vi "find lookahead point.vi"(6 "Lookahead Distance":dbl=4000.0, 11 "Path Data":T1={"Path"=[], "Target Velocities"=[], "Robot Location"=[], "Relative Robot Angle (rad)"=0.0, "Curvature"=0.0, "Lookahead Point"=[3064.399009129367, 18229.833030071386], "Lookahead Index"=8.422809037111724, "Closest Point"=[], "Closest Point Index"=0, "Left Velocity"=0.0, "Right Velocity"=0.0, "Left Encoder Vel"=0, "Right Encoder Vel"=0, "Left Encoder Pos"=0, "Right Encoder Pos"=0, "Inital Robot Angle (deg)"=0.0}) -> (3 "Path Data":T1={"Path"=[], "Target Velocities"=[], "Robot Location"=[], "Relative Robot Angle (rad)"=0.0, "Curvature"=0.0, "Lookahead Point"=[3064.399009129367, 18229.833030071386], "Lookahead Index"=8.422809037111724, "Closest Point"=[], "Closest Point Index"=0, "Left Velocity"=0.0, "Right Velocity"=0.0, "Left Encoder Vel"=0, "Right Encoder Vel"=0, "Left Encoder Pos"=0, "Right Encoder Pos"=0, "Inital Robot Angle (deg)"=0.0})   [LabVIEW 2018]
uses:
  path data.ctl
panel:
  out "a":dbl
  out "Lookahead Index":dbl=8.422809037111724
  out "Lookahead Point":dbl[](array[numeric])=[3064.399009129367, 18229.833030071386]
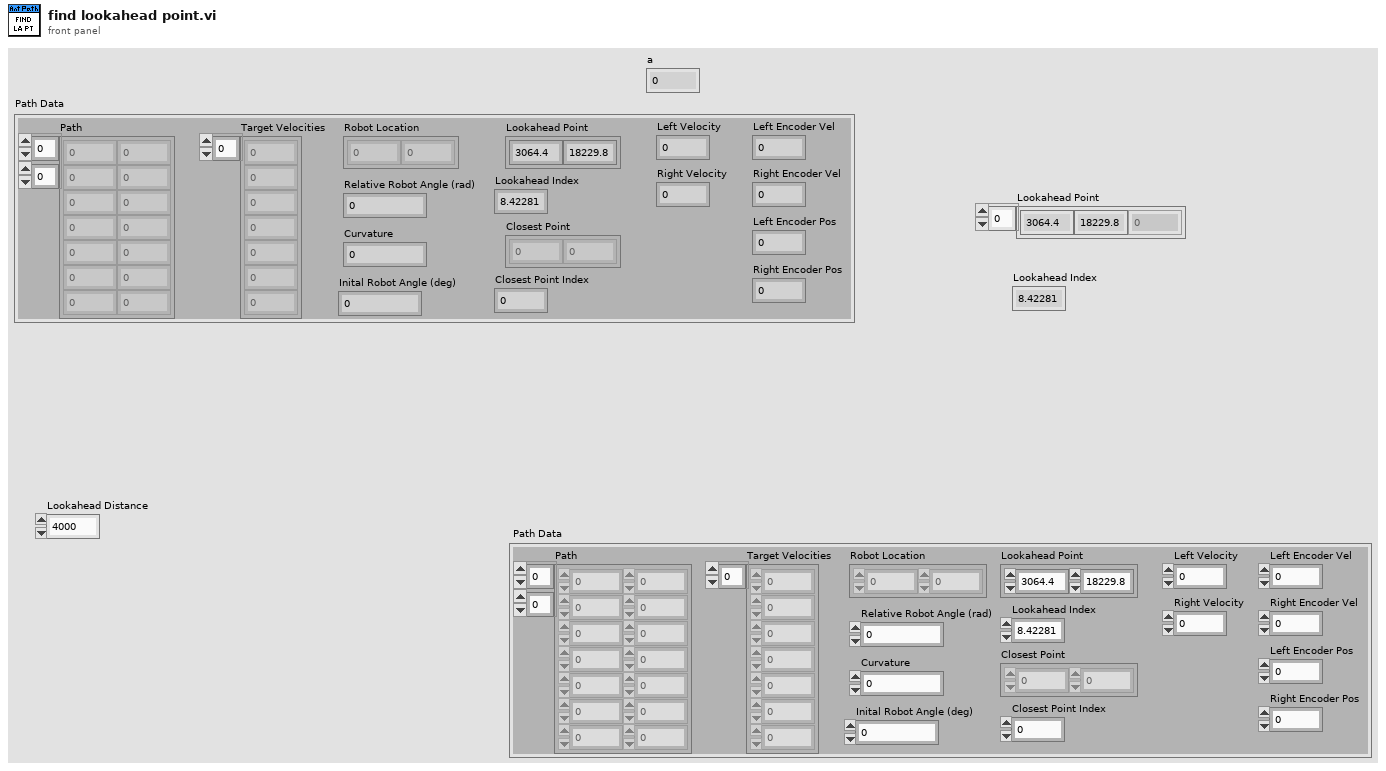
[diagram p1: front panel]
types:
  T1 = typedef "path data.ctl" = cluster{"Path":dbl[][], "Target Velocities":dbl[], "Robot Location":dbl[], "Relative Robot Angle (rad)":dbl, "Curvature":dbl, "Lookahead Point":dbl[], "Lookahead Index":dbl, "Closest Point":dbl[], "Closest Point Index":i32, "Left Velocity":dbl, "Right Velocity":dbl, "Left Encoder Vel":i32, "Right Encoder Vel":i32, "Left Encoder Pos":i32, "Right Encoder Pos":i32, "Inital Robot Angle (deg)":dbl}
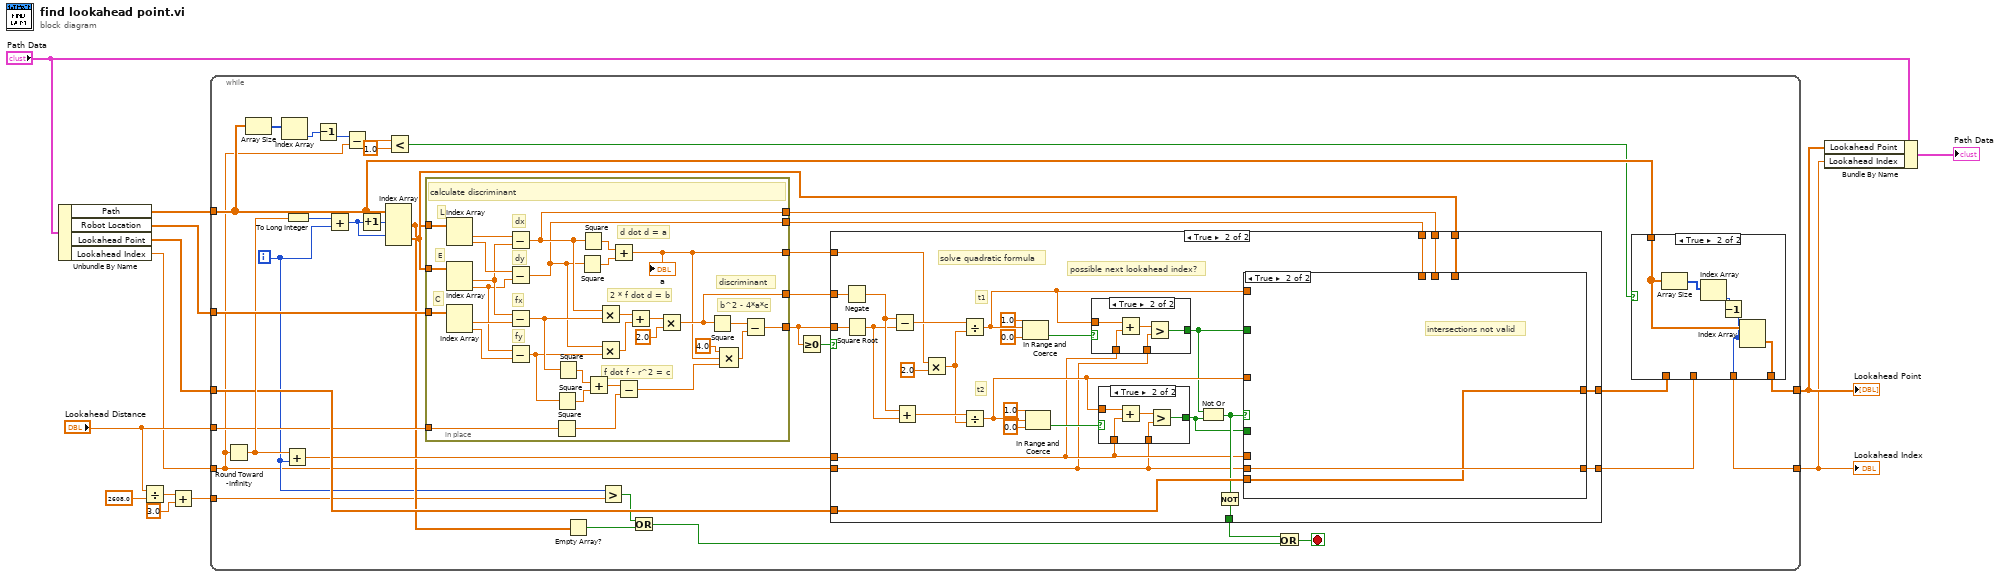
[diagram p0: block diagram]
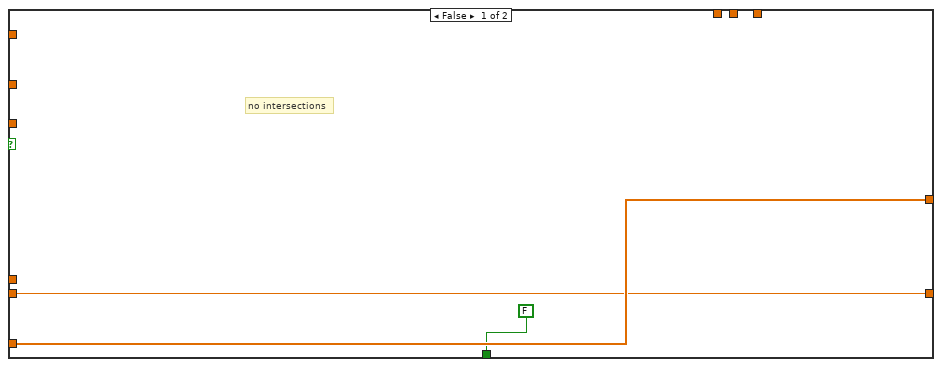
[diagram p3: hidden frame]
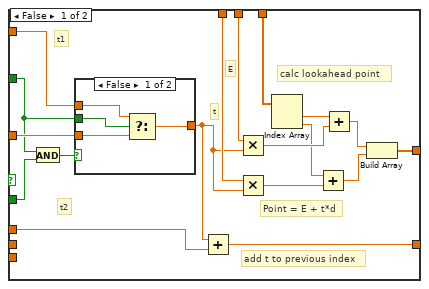
[diagram p4: hidden frame]
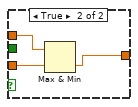
[diagram p5: hidden frame]
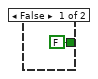
[diagram p6: hidden frame]
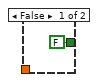
[diagram p7: hidden frame]
diagram:
  n1 = Unbundle By Name("Path Data") -> ("Path"=w4:dbl[][], "Robot Location"=w3:dbl[], "Lookahead Point"=w2:dbl[], "Lookahead Index"=w1:dbl)
  n2 = Divide(x="Lookahead Distance", y=2608.0) -> (x/y=w11:dbl)
  n3 = Add(x=w11, y=3.0) -> (x+y=w9:dbl)
  n4 = while {
    tunnel: w3 -> [w48]
    tunnel: "Lookahead Distance" -> [w39]
    tunnel: w4 -> [w25]
    tunnel: w1 -> [w23]
    tunnel: w2 -> [w41]
    tunnel: [w18] -> w6
    tunnel: [w16] -> w5
    tunnel: w9 -> [w27]
    i -> [w28]
    stop <- w37 stop-if-true
    n5 = Round Toward -Infinity(1:w23) -> (0:w42:dbl)
    n6 = Array Size(array=w25) -> (size(s)=w24:i32[])
    n7 = Index Array(array=w24) -> (element=w15:i32)  [unwired: 1 in]
    n8 = Add(x=w42, y=w28) -> (x+y=w35:dbl)
    n9 = To Long Integer(number=w42) -> (32bit integer=w40:i32)
    n10 = Decrement(x=w15) -> (x-1=w14:i32)
    n11 = Add(x=w40, y=w28) -> (x+y=w34:i32)
    n12 = Subtract(x=w14, y=w23) -> (x-y=w22:dbl)
    n13 = Increment(x=w34) -> (x+1=w32:i32)
    n14 = Index Array(array=w25, index (row) #1=w32, index (row) #2=w34) -> (element #1=w31:dbl[], element #2=w33:dbl[])  [unwired: 2 in]
    n15 = Less?(x=w22, y=1.0) -> (x < y?=w20:bool)
    n16 = in-place {
      in-place-border: w48 -> [w86]
      in-place-border: w39 -> [w69]
      in-place-border: [w62] -> w47
      in-place-border: [w61] -> w46
      in-place-border: [w60] -> w45
      in-place-border: [w59] -> w44
      in-place-border: [w58] -> w43
      in-place-border: w31 -> [w57]
      in-place-border: w33 -> [w56]
      # "C"
      # "E"
      # "L"
      # "calculate discriminant"
      # "b^2 - 4*a*c"
      # "discriminant"
      # "f dot f - r^2 = c"
      # "2 * f dot d = b"
      # "d dot d = a"
      # "fy"
      # "dy"
      # "fx"
      # "dx"
      n17 = Index Array(array=w57) -> (element #1=w85:dbl, element #2=w84:dbl)  [unwired: 2 in]
      n18 = Index Array(array=w56) -> (element #1=w83:dbl, element #2=w81:dbl)  [unwired: 2 in]
      n19 = Index Array(array=w86) -> (element #1=w82:dbl, element #2=w80:dbl)  [unwired: 2 in]
      n20 = Subtract(x=w85, y=w83) -> (x-y=w60:dbl)
      n21 = Subtract(x=w84, y=w81) -> (x-y=w59:dbl)
      n22 = Subtract(x=w83, y=w82) -> (x-y=w73:dbl)
      n23 = Subtract(x=w81, y=w80) -> (x-y=w72:dbl)
      n24 = Square(x=w69) -> (x^2=w68:dbl)
      n25 = Square(x=w72) -> (x^2=w70:dbl)
      n26 = Square(x=w73) -> (x^2=w71:dbl)
      n27 = Square(x=w59) -> (x^2=w79:dbl)
      n28 = Square(x=w60) -> (x^2=w78:dbl)
      n29 = Add(x=w71, y=w70) -> (x+y=w67:dbl)
      n30 = Multiply(x=w60, y=w73) -> (x*y=w77:dbl)
      n31 = Multiply(x=w59, y=w72) -> (x*y=w76:dbl)
      n32 = Add(x=w78, y=w79) -> (x+y=w58:dbl)
      "a" <- w58
      n33 = Subtract(x=w67, y=w68) -> (x-y=w64:dbl)
      n34 = Add(x=w77, y=w76) -> (x+y=w75:dbl)
      n35 = Multiply(x=w75, y=2.0) -> (x*y=w62:dbl)
      n36 = Square(x=w62) -> (x^2=w66:dbl)
      n37 = Compound Arithmetic op=MULTIPLY(4.0 ("value"), w58, w64) -> (w63:dbl)
      n38 = Subtract(x=w66, y=w63) -> (x-y=w61:dbl)
    }
    n39 = Empty Array?(array=w31) -> (empty?=w30:bool)
    n40 = Greater?(x=w28, y=w27) -> (0:w26:bool)
    n41 = Or(x=w26, y=w30) -> (x .or. y?=w29:bool)
    n42 = Greater Or Equal To 0?(x=w46) -> (x >= 0?=w36:bool)
    n43 = case shown="True" w36 {
      tunnel: w41 -> [w89 w104]
      tunnel: [w89 w103] -> w19
      tunnel: w47 -> [_ w112]
      tunnel: w43 -> [_ w99]
      tunnel: w46 -> [_ w111]
      tunnel: w35 -> [_ w91]
      tunnel: w33 -> [_ w102]
      tunnel: w45 -> [_ w101]
      tunnel: w44 -> [_ w100]
      tunnel: w23 -> [w87 w90]
      tunnel: [FALSE w95] -> w38
      tunnel: [w87 w92] -> w17
      frame False {
        # "no intersections"
      }
      frame True {
        # "solve quadratic formula"
        # "possible next lookahead index?"
        # "t2"
        # "t1"
        n44 = Negate(x=w112) -> (-x=w116:dbl)
        n45 = Square Root(x=w111) -> (sqrt(x)=w115:dbl)
        n46 = Subtract(x=w116, y=w115) -> (x-y=w117:dbl)
        n47 = Add(x=w116, y=w115) -> (x+y=w114:dbl)
        n48 = Multiply(x=w99, y=2.0) -> (x*y=w113:dbl)
        n49 = Divide(x=w117, y=w113) -> (x/y=w98:dbl)
        n50 = Divide(x=w114, y=w113) -> (x/y=w97:dbl)
        n51 = In Range and Coerce(upper limit=1.0, x=w98, lower limit=0.0) -> (In Range?=w105:bool)  [unwired: 1 out]
        n52 = In Range and Coerce(upper limit=1.0, x=w97, lower limit=0.0) -> (In Range?=w106:bool)  [unwired: 1 out]
        n53 = case shown="True" w105 {
          tunnel: w98 -> [_ w151]
          tunnel: w91 -> [_ w150]
          tunnel: w90 -> [_ w148]
          tunnel: [FALSE w147] -> w94
          frame False {
          }
          frame True {
            n54 = Add(x=w151, y=w150) -> (x+y=w149:dbl)
            n55 = Greater?(x=w149, y=w148) -> (0:w147:bool)
          }
        }
        n56 = case shown="True" w106 {
          tunnel: w97 -> [_ w157]
          tunnel: w91 -> [_ w156]
          tunnel: w90 -> [_ w154]
          tunnel: [FALSE w153] -> w93
          frame False {
          }
          frame True {
            n57 = Add(x=w157, y=w156) -> (x+y=w155:dbl)
            n58 = Greater?(x=w155, y=w154) -> (0:w153:bool)
          }
        }
        n59 = Not Or(1:w93, 2:w94) -> (0:w96:bool)
        n60 = Not(x=w96) -> (.not. x?=w95:bool)
        n61 = case shown="True" w96 {
          tunnel: w98 -> [w134 _]
          tunnel: w97 -> [w133 _]
          tunnel: w104 -> [_ w144]
          tunnel: [w122 w144] -> w103
          tunnel: w94 -> [w132 _]
          tunnel: w93 -> [w136 _]
          tunnel: w102 -> [w125 _]
          tunnel: w101 -> [w124 _]
          tunnel: w100 -> [w123 _]
          tunnel: [w120 w145] -> w92
          tunnel: w91 -> [w119 _]
          tunnel: w90 -> [_ w145]
          frame False {
            # "add t to previous index"
            # "Point = E + t*d"
            # "calc lookahead point"
            # "t"
            # "t2"
            # "t1"
            # "E"
            n62 = And(x=w132, y=w136) -> (x .and. y?=w135:bool)
            n63 = case shown="False" w135 {
              tunnel: w134 -> [w139 w143]
              tunnel: w133 -> [w138 w142]
              tunnel: [w137 w141] -> w121
              tunnel: w132 -> [w140 _]
              frame False {
                n64 = Select(t=w139, s=w140, f=w138) -> (s? t:f=w137:dbl)
              }
              frame True {
                n65 = Max & Min(x=w143, y=w142) -> (min(x,y)=w141:dbl)  [unwired: 1 out]
              }
            }
            n66 = Add(x=w121, y=w119) -> (x+y=w120:dbl)
            n67 = Multiply(x=w124, y=w121) -> (x*y=w129:dbl)
            n68 = Multiply(x=w123, y=w121) -> (x*y=w128:dbl)
            n69 = Index Array(array=w125) -> (element #1=w127:dbl, element #2=w126:dbl)  [unwired: 2 in]
            n70 = Add(x=w126, y=w128) -> (x+y=w130:dbl)
            n71 = Add(x=w127, y=w129) -> (x+y=w131:dbl)
            n72 = Build Array(w131, w130) -> (w122:dbl[])
          }
          frame True {
            # "intersections not valid"
          }
        }
      }
    }
    n73 = Or(x=w38, y=w29) -> (x .or. y?=w37:bool)
    n74 = case shown="True" w20 {
      tunnel: w25 -> [_ w53]
      tunnel: [w50 w52] -> w18
      tunnel: w19 -> [w50 _]
      tunnel: [w49 w51] -> w16
      tunnel: w17 -> [w49 _]
      frame False {
      }
      frame True {
        n75 = Array Size(array=w53) -> (size(s)=w54:i32[])
        n76 = Index Array(array=w54) -> (element=w55:i32)  [unwired: 1 in]
        n77 = Decrement(x=w55) -> (x-1=w51:i32)
        n78 = Index Array(array=w53, index (row)=w51) -> (element=w52:dbl[])  [unwired: 1 in]
      }
    }
  }
  "Lookahead Point" <- w6
  "Lookahead Index" <- w5
  n79 = Bundle By Name(cluster="Path Data", "Lookahead Point"=w6, "Lookahead Index"=w5) -> (→"Path Data":T1)
